vi "Abs-Path.vi"(10 "filename":path, 11 "Vi in path":refnum<vi>) -> (3 "Full path":path)   [LabVIEW 2017]
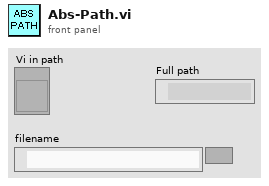
[diagram p1: front panel]
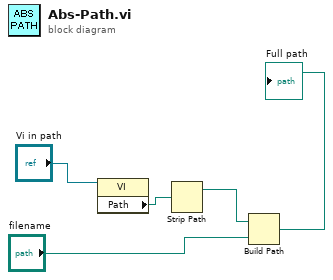
[diagram p0: block diagram]
diagram:
  n1 = property class="VI"(reference="Vi in path") -> ("Path"=w3:path)  [unwired: 1 in, 2 out]
  n2 = Strip Path(path=w3) -> (stripped path=w4:path)  [unwired: 1 out]
  n3 = Build Path(base path=w4, name or relative path="filename") -> (appended path=→"Full path":path)
